vi "GetTabReference.vi"(8 "error in":errorcluster, 11 "Tab in":refnum<class "Tab.lvclass">) -> (0 "error out":errorcluster, 1 "tab reference":refnum<vi>, 3 "Tab out":refnum<class "Tab.lvclass">)   [LabVIEW 2014, in "Raspberry Pi Compatible Compiler for LabVIEW.lvlib" / "Tab.lvclass"]
uses:
  Tab.lvclass
  Generic/Generic.lvclass
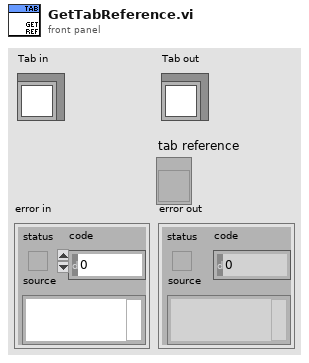
[diagram p1: front panel]
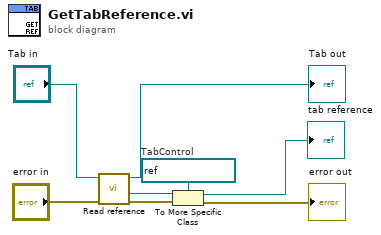
[diagram p0: block diagram]
diagram:
  w8 = refnum<vi> refnum  # TabControl
  n1 = call "Read reference.vi"("error in"="error in", "GObject in"="Tab in") -> ("error out"=w2:errorcluster, "reference"=w3:refnum<vi>, "GObject out"=→"Tab out":refnum<class "Tab.lvclass">)  [unwired: 5 in]
  n2 = To More Specific Class(target class=w8, reference=w3, error in=w2) -> (specific class reference=→"tab reference":refnum<vi>, error out=→"error out":errorcluster)
